vi "updateTestParameters.vi"(8 "error in (no error)":errorcluster, 11 "Model in":refnum<class "Model.lvclass">) -> (0 "error out":errorcluster, 3 "Model out":refnum<class "Model.lvclass">)   [LabVIEW 2013, in "Model.lvclass"]
uses:
  Model.lvclass
  Configuration/TestParameters.ctl
  Configuration/CycleProfileConfig.ctl
  Model.lvclass/Model.ctl
  ApplicationElements/TestMonitor/TestMonitor.lvclass/TestMonitor.ctl
  ApplicationElements/TestMonitor/TestMonitor.lvclass
  ConfigurationThisComponent/ConfigurationThisComponent.lvclass
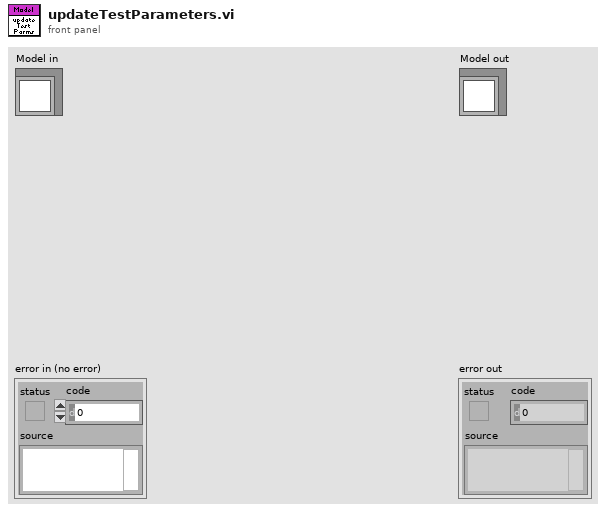
[diagram p1: front panel]
types:
  T1 = typedef "TestParameters.ctl" = cluster{"Number of cycles for complete test":u32, "Cycle profile":T2, "PGA Gain Coefficients":u8[], "Temperature Transition Wait Time":dbl[unit], "Temperature Settled StDev":dbl[unit], "Temperature Settling Sample Size":u16, "Bridge Measurement Sample Size":u16}
  T2 = typedef "CycleProfileConfig.ctl" = cluster{"Temperature Setpoint":dbl[unit][], "Soak Time":dbl[unit][], "Gain Stabilization Time":dbl[unit][], "Pause After Step":dbl[unit][]}
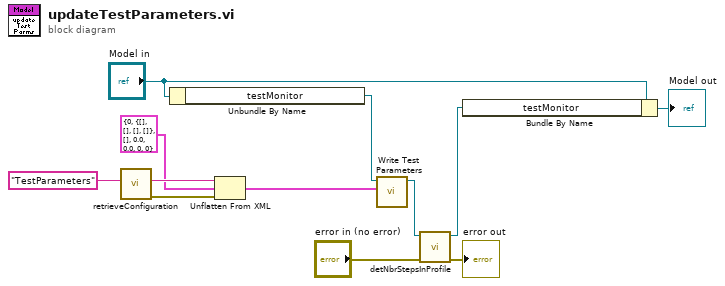
[diagram p0: block diagram]
diagram:
  n1 = call "retrieveConfiguration.vi"("configName"="TestParameters") -> ("error out"=w4:errorcluster, "xmlConfig"=w3:string)  [unwired: 8 in, 1 out]
  n2 = Unbundle By Name("Model in") -> ("testMonitor"=w11:refnum<class "TestMonitor.lvclass">)
  n3 = Unflatten From XML(xml string=w3, type=T1 {"Number of cycles for complete test"=0, "Cycle profile"={"Temperature Setpoint"=[], "Soak Time"=[], "Gain Stabilization Time"=[], "Pause After Step"=[]}, "PGA Gain Coefficients"=[], "Temperature Transition Wait Time"=0.0, "Temperature Settled StDev"=0.0, "Temperature Settling Sample Size"=0, "Bridge Measurement Sample Size"=0} ("Test Parameters"), error in (no error)=w4) -> (value=w1:T1)  [unwired: 1 out]
  n4 = call "Write Test Parameters.vi"("Test Parameters"=w1, "TestMonitor in"=w11) -> ("TestMonitor out"=w10:refnum<class "TestMonitor.lvclass">)  [unwired: 9 in]
  n5 = call "detNbrStepsInProfile.vi"("error in (no error)"="error in (no error)", "TestMonitor in"=w10) -> ("error out"=→"error out":errorcluster, "TestMonitor out"=w9:refnum<class "TestMonitor.lvclass">)  [unwired: 8 in]
  n6 = Bundle By Name(cluster="Model in", "testMonitor"=w9) -> (→"Model out":refnum<class "Model.lvclass">)
